vi "LOGGER Loop.vi"(8 "error in":errorcluster, 10 "Queues":T1, 11 "Notifiers":T2) -> (0 "error out":errorcluster)   [LabVIEW 2014, in "Logger.lvlib"]
uses:
  Logger.lvlib
  support/Message Queue/Message Queue.lvlib
  TypeDefs/Logger State.ctl
  TypeDefs/Logger Data.ctl
  Model/TypeDefs/Get Model Status Control.ctl
  Model/Model.lvlib
  <vilib>/ErrorRing/Error Ring.xnode
  support/Global names.vi
  <vilib>/Utility/error.llb/Error Cluster From Error Code.vi
  Report/Report.lvlib
  Report/TypeDefs/Report state.ctl
  support/Message Queue/Message Cluster.ctl
  support/Notifiers/Notifiers.ctl
  Support/Notifiers/Notifiers.lvlib
  support/Message Queue/All Message Queues.ctl
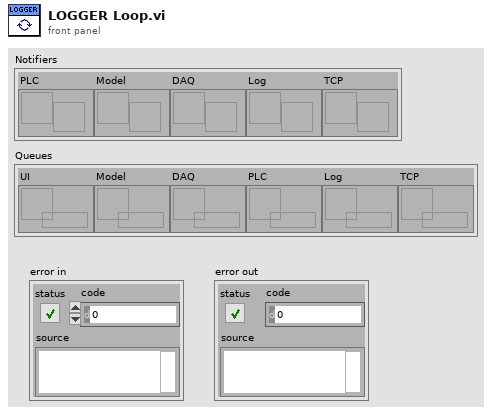
[diagram p1: front panel]
types:
  T1 = typedef "Message Queue.lvlib/All Message Queues.ctl" = cluster{"UI":refnum<queue>, "Model":refnum<queue>, "DAQ":refnum<queue>, "PLC":refnum<queue>, "Log":refnum<queue>, "TCP":refnum<queue>}
  T2 = typedef "Notifiers.lvlib/Notifiers.ctl" = cluster{"PLC":refnum<notifier>, "Model":refnum<notifier>, "DAQ":refnum<notifier>, "Log":refnum<notifier>, "TCP":refnum<notifier>}
  T3 = typedef "Logger.lvlib/Logger Data.ctl" = cluster{"tdms file out":refnum<k34>, "State":T4, "Path":path}
  T4 = typedef "Logger.lvlib/Logger State.ctl" = enum16{"Idle", "Working"}
  T5 = typedef "Report.lvlib/Report state.ctl" = enum16{"Create report", "Save data", "Save report", "Available printers", "Print report", "Close report"}
  T6 = enum16{"open", "open or create", "create or replace", "create", "open (read-only)"}
  T7 = typedef "Model.lvlib/Get Model Status Control.ctl" = cluster{"Position":dbl, "Pump State":bool, "Fluid Flow":dbl, "Fluid Level":dbl, "Barrel Number":i32, "Spill Alarm":bool, "Level Alarm":bool}
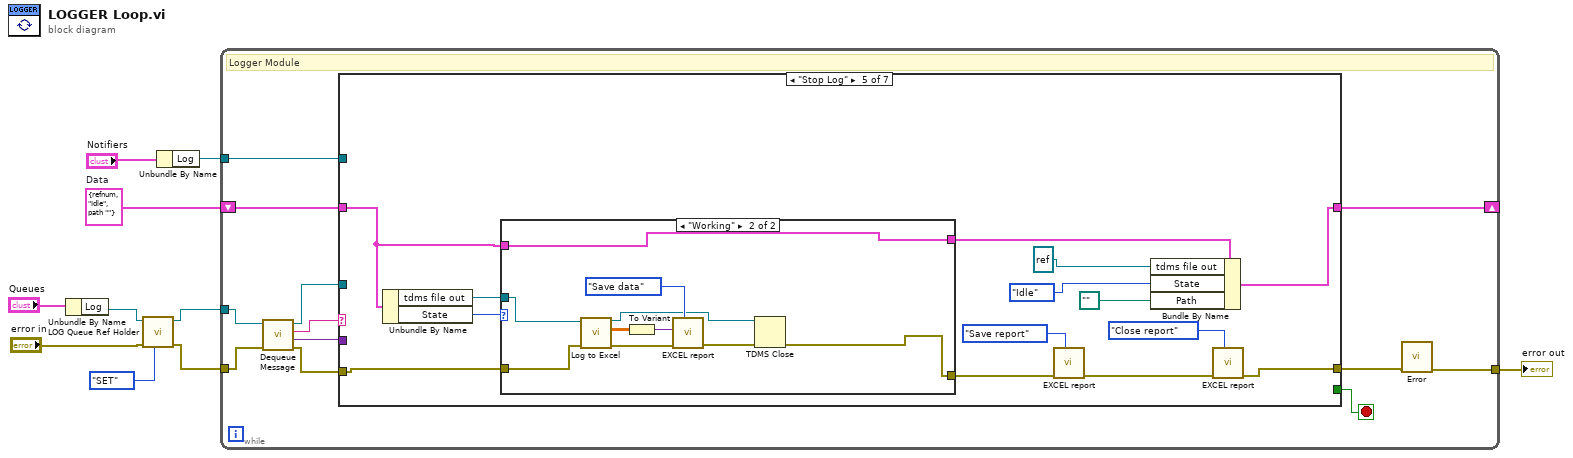
[diagram p0: block diagram]
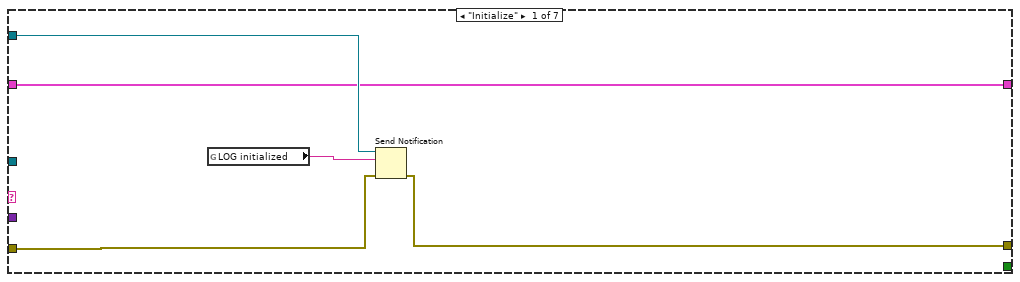
[diagram p2: hidden frame]
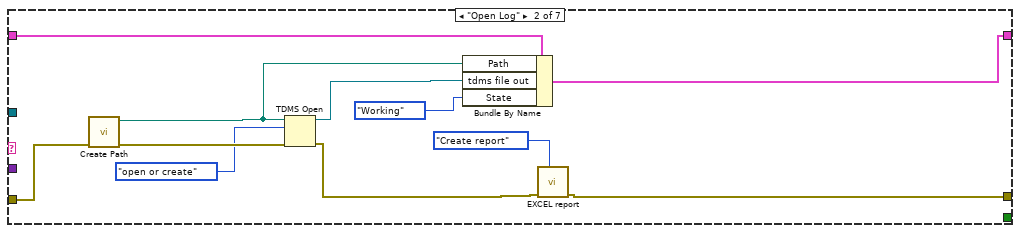
[diagram p3: hidden frame]
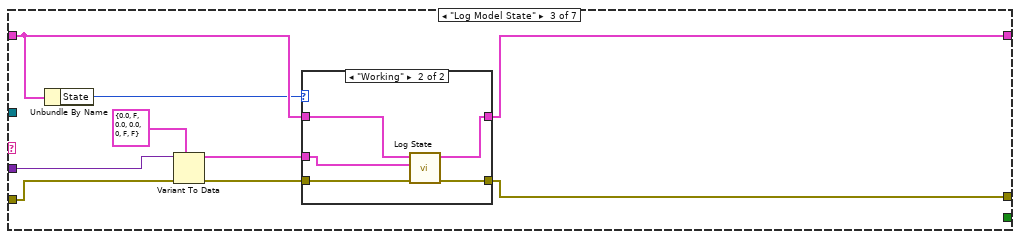
[diagram p4: hidden frame]
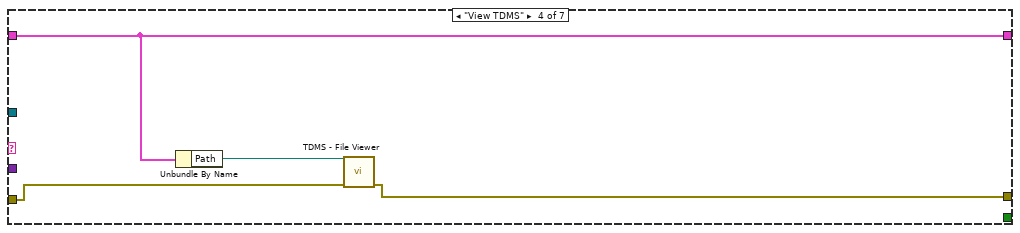
[diagram p6: hidden frame]
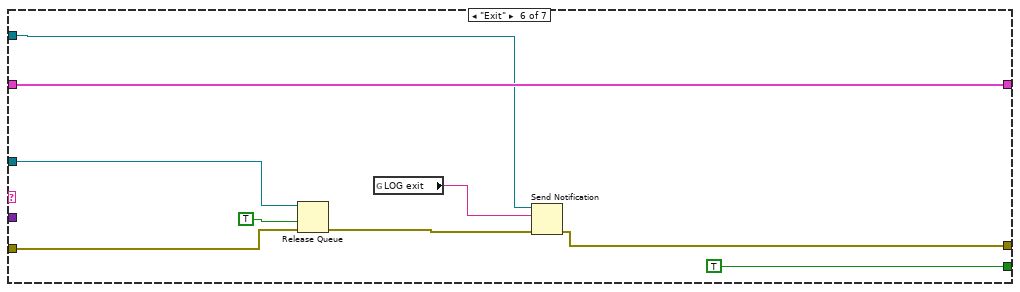
[diagram p8: hidden frame]
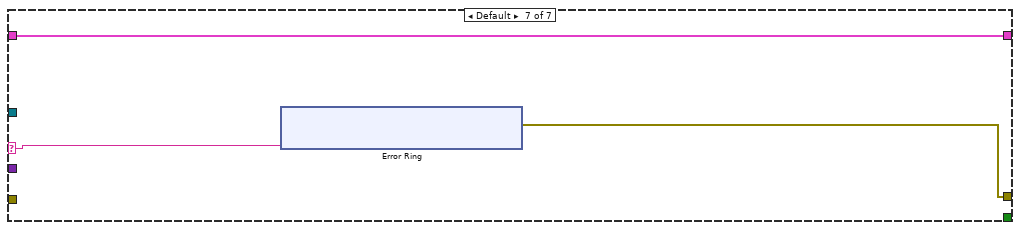
[diagram p9: hidden frame]
diagram:
  w10 = T3 {"tdms file out"=refnum, "State"=enum."Idle", "Path"=path ""}  # Data
  n1 = Unbundle By Name("Queues") -> ("Log"=w3:refnum<queue>)
  n2 = call "LOG Queue Ref Holder.vi"("Action"=enum16{"GET", "SET"}."SET", "error in"="error in", "Message Queue In"=w3) -> ("error out"=w4:errorcluster, "Input Message Queue"=w2:refnum<queue>)  [unwired: 7 in]
  n3 = Unbundle By Name("Notifiers") -> ("Log"=w6:refnum<notifier>)
  n4 = while {
    tunnel: w4 -> [w22]
    tunnel: w2 -> [w21]
    tunnel: [w11] -> w9
    shift-right: [w14] -> _
    shift-left: w10 -> [w15]
    tunnel: w6 -> [w13]
    stop <- w16 stop-if-true
    # "Logger Module"
    n5 = call "Dequeue Message.vi"("error in (no error)"=w22, "Message Queue"=w21) -> ("error out"=w20:errorcluster, "Message Data"=w17:variant, "Message"=w19:string, "dup Message Queue"=w18:refnum<queue>)  [unwired: 6 in]
    n6 = case shown="\"Stop Log\"" w19 {
      selector: w19 -> [_ _ _ _ _ _ w95]
      tunnel: w20 -> [w24 w38 w47 w58 w68 w90 _]
      tunnel: w18 -> [_ _ _ _ _ w89 _]
      tunnel: w17 -> [_ _ w45 _ _ _ _]
      tunnel: [w25 w29 w42 w56 w61 w91 w94] -> w12
      tunnel: [_ _ _ _ _ TRUE _] -> w16
      tunnel: w15 -> [w26 w35 w40 w57 w65 w93 w96]
      tunnel: [w26 w31 w41 w57 w72 w93 w96] -> w14
      tunnel: w13 -> [w27 _ _ _ _ w86 _]
      frame "Initialize" {
        n7 = global read "Global names.vi" "LOG initialized"() -> (w23:string)
        n8 = Send Notification(notification=w23, notifier=w27, error in (no error)=w24) -> (error out=w25:errorcluster)  [unwired: 1 out]
      }
      frame "Open Log" {
        n9 = call "Create Path.vi"("error in (no error)"=w38) -> ("error out"=w37:errorcluster, "File Path Control"=w33:path)  [unwired: 9 in]
        n10 = TDMS Open(8:w37, 10:T6."open or create" ("operation (0:open)"), 11:w33) -> (0:w30:errorcluster, 3:w32:refnum<k34>)  [unwired: 4 in]
        n11 = Bundle By Name(cluster=w35, "Path"=w33, "tdms file out"=w32, "State"=Logger_State."Working") -> (w31:T3)
        n12 = call "EXCEL report.vi"("Report state"=Report_state."Create report", "error in"=w30) -> ("error out"=w29:errorcluster)  [unwired: 8 in, 1 out]
      }
      frame "Log Model State" {
        n13 = Unbundle By Name(w40) -> ("State"=w39:T4)
        n14 = Variant To Data(error in=w47, type=T7 {"Position"=0.0, "Pump State"=FALSE, "Fluid Flow"=0.0, "Fluid Level"=0.0, "Barrel Number"=0, "Spill Alarm"=FALSE, "Level Alarm"=FALSE} ("Model Status"), Variant=w45) -> (data=w44:T7, error out=w43:errorcluster)
        n15 = case shown="\"Working\"" w39 {
          tunnel: w44 -> [_ w54]
          tunnel: w43 -> [w48 w53]
          tunnel: [w48 w50] -> w42
          tunnel: [w49 w51] -> w41
          tunnel: w40 -> [w49 w52]
          frame Default {
          }
          frame "Working" {
            n16 = call "Log State.vi"("error in (no error)"=w53, "Model Status"=w54, "Data"=w52) -> ("error out"=w50:errorcluster, "Data out"=w51:T3)  [unwired: 7 in]
          }
        }
      }
      frame "View TDMS" {
        n17 = Unbundle By Name(w57) -> ("Path"=w55:path)
        n18 = call <vilib>:"TDMS - File Viewer.vi"("error in (no error)"=w58, "file path"=w55) -> ("error out"=w56:errorcluster)  [unwired: 4 in, 1 out]
      }
      frame "Stop Log" {
        n19 = Unbundle By Name(w65) -> ("tdms file out"=w69:refnum<k34>, "State"=w66:T4)
        n20 = case shown="\"Working\"" w66 {
          tunnel: w69 -> [_ w78]
          tunnel: w68 -> [w74 w83]
          tunnel: [w74 w76] -> w63
          tunnel: w65 -> [w73 w84]
          tunnel: [w73 w84] -> w64
          frame "Idle", Default {
          }
          frame "Working" {
            n21 = call "Log to Excel.vi"("error in"=w83, "tdms file in"=w78) -> ("error out"=w82:errorcluster, "appended array"=w81:dbl[][][], "tdms file out"=w75:refnum<k34>)  [unwired: 7 in]
            n22 = To Variant(anything=w81) -> (Variant=w80:variant)
            n23 = call "EXCEL report.vi"("Report state"=Report_state."Save data", "error in"=w82, "Data in"=w80) -> ("error out"=w77:errorcluster)  [unwired: 7 in, 1 out]
            n24 = TDMS Close(8:w77, 11:w75) -> (0:w76:errorcluster)  [unwired: 1 out]
          }
        }
        n25 = call "EXCEL report.vi"("Report state"=Report_state."Save report", "error in"=w63) -> ("error out"=w62:errorcluster)  [unwired: 8 in, 1 out]
        n26 = Bundle By Name(cluster=w64, "tdms file out"=refnum<k34> refnum, "State"=Logger_State."Idle", "Path"=path "") -> (w72:T3)
        n27 = call "EXCEL report.vi"("Report state"=Report_state."Close report", "error in"=w62) -> ("error out"=w61:errorcluster)  [unwired: 8 in, 1 out]
      }
      frame "Exit" {
        n28 = Release Queue(queue=w89, force destroy? (F)=TRUE, error in (no error)=w90) -> (error out=w88:errorcluster)  [unwired: 2 out]
        n29 = global read "Global names.vi" "LOG exit"() -> (w85:string)
        n30 = Send Notification(notification=w85, notifier=w86, error in (no error)=w88) -> (error out=w91:errorcluster)  [unwired: 1 out]
      }
      frame Default {
        n31 = xnode "Error Ring"("parameter 0"=w95) -> ("error out"=w94:errorcluster)
      }
    }
    n32 = call "Error.vi"("error in"=w12) -> ("error out"=w11:errorcluster)  [unwired: 10 in]
  }
  "error out" <- w9
